vi "My Check Fit Convergence.vi"(0 "Chi 2":dbl, 1 "Lambda":dbl=-1.0, 5 "Parameters":dbl[](array[numeric]), 7 "gradient":dbl[](array[numeric]), 9 "my stopping criteria":T2={"Max Iterations"=0, "Max Function Calls"=0, "Max Time"=1000.0, "Function Tolerance"=1e-06, "Parameter Tolerance"=1e-06, "Gradient Tolerance"=0.0, "Min Lambda"=1e-06, "Max Lambda"=1e-06, "Initial Tick Count"=0} {"Max Time" min=-2147483648.0 max=2147483647.0}, 11 "Error In":errorcluster, 12 "current iteration":i32, 13 "number of function evaluations":i32) -> (2 "Gradient":dbl, 3 "|Delta Chi 2|/Chi 2":dbl, 4 "stop?":bool, 6 "|Delta Chi 2|":dbl, 8 "Max |Delta a| /|a|":dbl, 10 "Lambda":dbl=-1.0, 14 "Convergence Criterium Reached":T1, 15 "error out":errorcluster)   [LabVIEW 2021, in "Fits.lvlib"]
uses:
  Fits.lvlib
  My Fit Stopping Criteria.ctl
  Convergence Criteria.ctl
  <vilib>/Utility/error.llb/Error Cluster From Error Code.vi
  <vilib>/ErrorRing/Error Ring.xnode
  Error/Error.lvlib
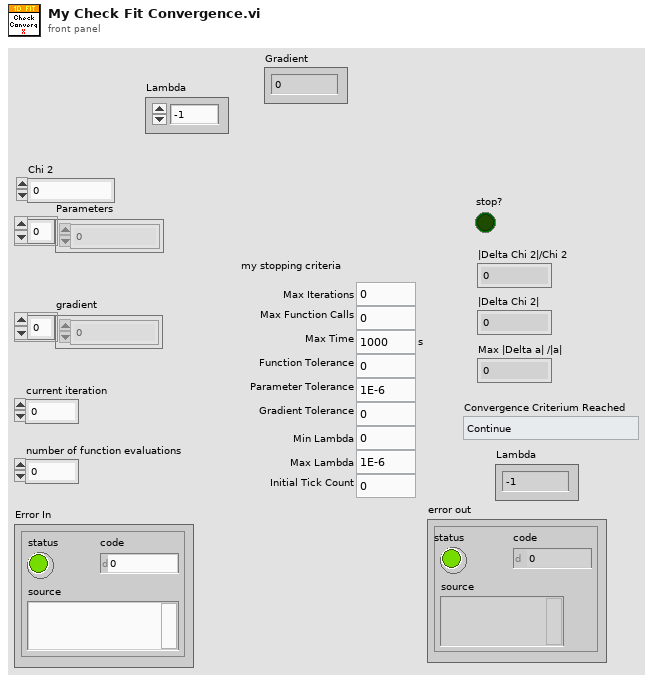
[diagram p1: front panel]
types:
  T1 = typedef "Fits.lvlib/Convergence Criteria.ctl" = enum16{"Continue", "Tolerances Exceeded", "Max Time Exceeded", "Max Iterations Exceeded", "Max Function Evaluations Exceeded", "Scale Range Exceeded"}
  T2 = typedef "Fits.lvlib/My Fit Stopping Criteria.ctl" = cluster{"Max Iterations":i32, "Max Function Calls":i32, "Max Time":dbl[unit], "Function Tolerance":dbl, "Parameter Tolerance":dbl, "Gradient Tolerance":dbl, "Min Lambda":dbl, "Max Lambda":dbl, "Initial Tick Count":u32}
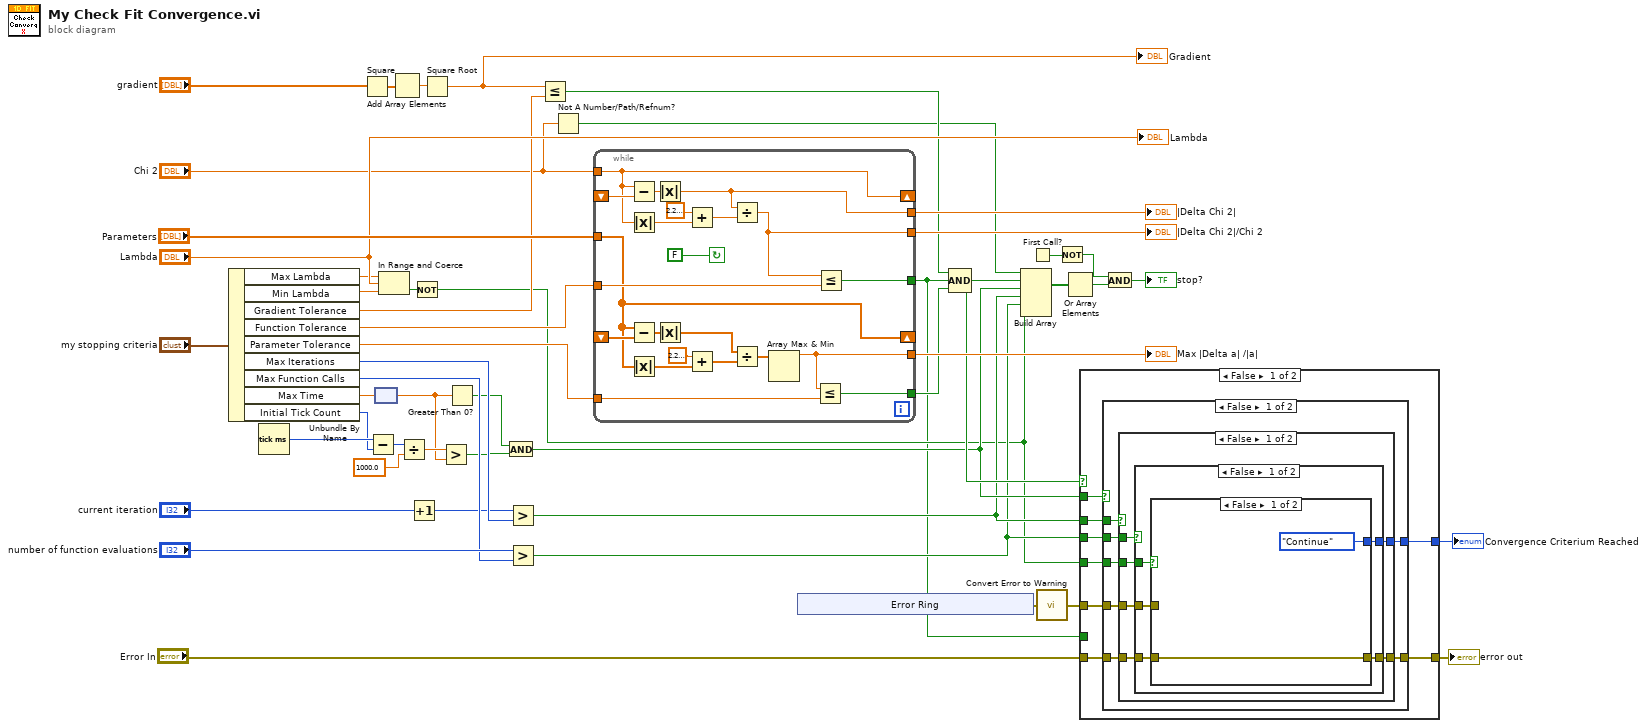
[diagram p0: block diagram]
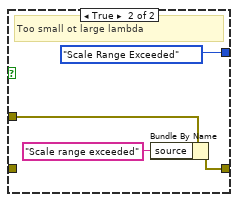
[diagram p2: hidden frame]
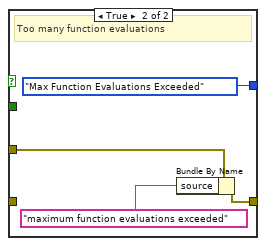
[diagram p3: hidden frame]
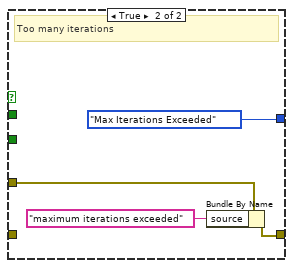
[diagram p4: hidden frame]
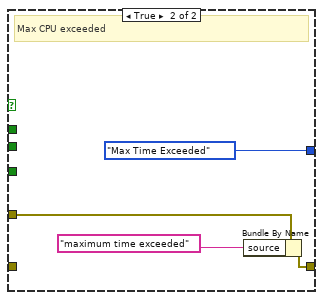
[diagram p5: hidden frame]
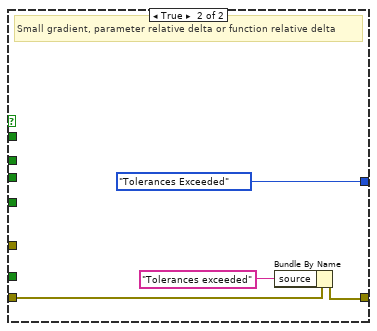
[diagram p6: hidden frame]
diagram:
  n1 = Unbundle By Name("my stopping criteria") -> ("Max Lambda"=w19:dbl, "Min Lambda"=w18:dbl, "Gradient Tolerance"=w29:dbl, "Function Tolerance"=w39:dbl, "Parameter Tolerance"=w38:dbl, "Max Iterations"=w37:i32, "Max Function Calls"=w36:i32, "Max Time"=w21:dbl[unit], "Initial Tick Count"=w25:u32)
  n2 = Tick Count (ms)() -> (millisecond timer value=w26:u32)
  n3 = Square(x="gradient") -> (x^2=w32:dbl[])
  n4 = Subtract(x=w26, y=w25) -> (x-y=w24:u32)
  n5 = node(w21) -> (w16:dbl)
  n6 = In Range and Coerce(upper limit=w19, x="Lambda", lower limit=w18) -> (In Range?=w17:bool)  [unwired: 1 out]
  n7 = Add Array Elements(numeric array=w32) -> (sum=w31:dbl)
  n8 = Divide(x=w24, y=1000.0) -> (x/y=w22:dbl)
  n9 = Increment(x="current iteration") -> (x+1=w33:i32)
  n10 = Not(x=w17) -> (.not. x?=w9:bool)
  n11 = Square Root(x=w31) -> (sqrt(x)=w30:dbl)
  "Gradient" <- w30
  n12 = Greater?(x=w22, y=w16) -> (0:w20:bool)
  n13 = Greater Than 0?(x=w16) -> (x > 0?=w27:bool)
  n14 = And(x=w27, y=w20) -> (x .and. y?=w12:bool)
  n15 = Greater?(x=w33, y=w37) -> (0:w11:bool)
  n16 = Greater?(x="number of function evaluations", y=w36) -> (0:w10:bool)
  n17 = Less Or Equal?(x=w30, y=w29) -> (x <= y?=w28:bool)
  n18 = Not A Number/Path/Refnum?(number/path/refnum="Chi 2") -> (NaN/Path/Refnum?=w3:bool)
  n19 = while {
    shift-right: [w68] -> _
    shift-left: _ -> [w69]
    tunnel: "Chi 2" -> [w68]
    tunnel: [w52] -> w6
    tunnel: "Parameters" -> [w51]
    shift-right: [w51] -> _
    shift-left: _ -> [w71]
    tunnel: [w53] -> w40
    tunnel: w39 -> [w58]
    tunnel: w38 -> [w57]
    tunnel: [w60] -> w45
    tunnel: [w70] -> w44
    tunnel: [w54] -> w43
    stop <- FALSE continue-if-true
    n20 = Subtract(x=w68, y=w69) -> (x-y=w61:dbl)
    n21 = Absolute Value(x=w68) -> (abs(x)=w67:dbl)
    n22 = Subtract(x=w51, y=w71) -> (x-y=w62:dbl[])
    n23 = Absolute Value(x=w51) -> (abs(x)=w65:dbl[])
    n24 = Absolute Value(x=w61) -> (abs(x)=w60:dbl)
    n25 = Absolute Value(x=w62) -> (abs(x)=w59:dbl[])
    n26 = Add(x=2.220446049250313e-16 ("machine eps"), y=w67) -> (x+y=w66:dbl)
    n27 = Add(x=2.220446049250313e-16 ("machine eps"), y=w65) -> (x+y=w64:dbl[])
    n28 = Divide(x=w60, y=w66) -> (x/y=w54:dbl)
    n29 = Divide(x=w59, y=w64) -> (x/y=w63:dbl[])
    n30 = Array Max & Min(array=w63) -> (max value=w70:dbl)  [unwired: 3 out]
    n31 = Less Or Equal?(x=w70, y=w57) -> (x <= y?=w53:bool)
    n32 = Less Or Equal?(x=w54, y=w58) -> (x <= y?=w52:bool)
  }
  "|Delta Chi 2|" <- w45
  "Max |Delta a| /|a|" <- w44
  "|Delta Chi 2|/Chi 2" <- w43
  n33 = xnode "Error Ring"() -> ("error out"=w2:errorcluster)
  n34 = Compound Arithmetic op=AND(w28, w6, w40) -> (w13:bool)
  n35 = Build Array(w3, w13, w12, w11, w10, w9) -> (w14:bool[])
  n36 = First Call?() -> (First Call?: T/F=w35:bool)
  n37 = call "Convert Error to Warning.vi"("Error In"=w2) -> ("no Error Out"=w1:errorcluster)  [unwired: 8 in]
  n38 = Not(x=w35) -> (.not. x?=w34:bool)
  n39 = Or Array Elements(Boolean array=w14) -> (logical OR=w15:bool)
  n40 = case shown="False" w13 {
    tunnel: [w79 Convergence_Criteria."Tolerances Exceeded"] -> w8
    tunnel: w12 -> [w80 _]
    tunnel: w11 -> [w78 _]
    tunnel: w10 -> [w77 _]
    tunnel: w9 -> [w76 _]
    tunnel: "Error In" -> [w75 w117]
    tunnel: [w74 w118] -> w7
    tunnel: w6 -> [_ _]
    tunnel: w1 -> [w73 _]
    frame False {
      n41 = case shown="False" w80 {
        tunnel: [w86 Convergence_Criteria."Max Time Exceeded"] -> w79
        tunnel: w78 -> [w87 _]
        tunnel: w77 -> [w85 _]
        tunnel: w76 -> [w84 _]
        tunnel: w75 -> [w83 _]
        tunnel: [w82 w115] -> w74
        tunnel: w73 -> [w81 w113]
        frame False {
          n42 = case shown="False" w87 {
            tunnel: [w93 Convergence_Criteria."Max Iterations Exceeded"] -> w86
            tunnel: w85 -> [w92 _]
            tunnel: w84 -> [w91 _]
            tunnel: w83 -> [w90 _]
            tunnel: [w89 w111] -> w82
            tunnel: w81 -> [w88 w109]
            frame False {
              n43 = case shown="False" w92 {
                tunnel: [w97 Convergence_Criteria."Max Function Evaluations Exceeded"] -> w93
                tunnel: w91 -> [w98 _]
                tunnel: w90 -> [w96 _]
                tunnel: [w95 w107] -> w89
                tunnel: w88 -> [w94 w105]
                frame False {
                  n44 = case shown="False" w98 {
                    tunnel: [Convergence_Criteria."Continue" Convergence_Criteria."Scale Range Exceeded"] -> w97
                    tunnel: w96 -> [w99 _]
                    tunnel: [w99 w103] -> w95
                    tunnel: w94 -> [_ w101]
                    frame False {
                    }
                    frame True {
                      # "Too small ot large lambda"
                      n45 = Bundle By Name(cluster=w101, "source"="Scale range exceeded") -> (w103:errorcluster)
                    }
                  }
                }
                frame True {
                  # "Too many function evaluations"
                  n46 = Bundle By Name(cluster=w105, "source"="maximum function evaluations exceeded") -> (w107:errorcluster)
                }
              }
            }
            frame True {
              # "Too many iterations"
              n47 = Bundle By Name(cluster=w109, "source"="maximum iterations exceeded") -> (w111:errorcluster)
            }
          }
        }
        frame True {
          # "Max CPU exceeded"
          n48 = Bundle By Name(cluster=w113, "source"="maximum time exceeded") -> (w115:errorcluster)
        }
      }
    }
    frame True {
      # "Small gradient, parameter relative delta or function relative delta"
      n49 = Bundle By Name(cluster=w117, "source"="Tolerances exceeded") -> (w118:errorcluster)
    }
  }
  "error out" <- w7
  "Convergence Criterium Reached" <- w8
  n50 = And(x=w34, y=w15) -> (x .and. y?=→"stop?":bool)
  "Lambda" <- "Lambda"
